vi "Adjust Position.vi"(7 "VI in":refnum<vi>, 8 "error in":errorcluster, 11 "Current Position":T1) -> (0 "error out":errorcluster, 3 "Adjusted Position":T1)   [LabVIEW 2020, in "Editor Position.lvclass"]
doc: "Offsets to current windows bounds in order to prove the window was moved by the VI being tested."
uses:
  Editor Position.lvclass
  Editor Position.lvclass/Editor Position.ctl
  <vilib>/Utility/miscctls.llb/LVRectTypeDef.ctl
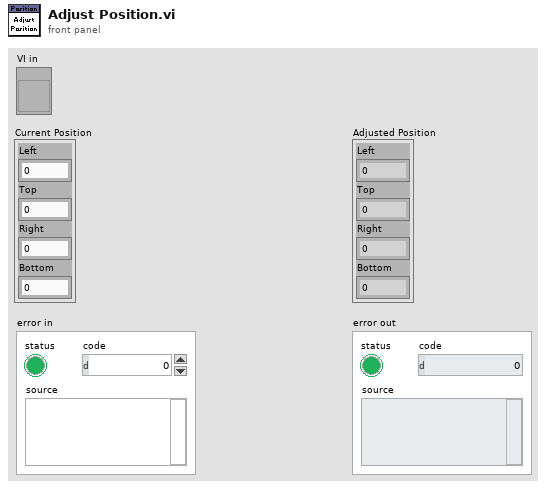
[diagram p1: front panel]
types:
  T1 = typedef "LVRectTypeDef.ctl" = cluster{"Left":i16, "Top":i16, "Right":i16, "Bottom":i16}
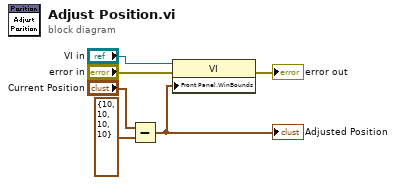
[diagram p0: block diagram]
diagram:
  n1 = Subtract(x="Current Position", y=T1 {"Left"=10, "Top"=10, "Right"=10, "Bottom"=10}) -> (x-y=w1:T1)
  "Adjusted Position" <- w1
  n2 = property class="VI"(reference="VI in", error in="error in", "Front Panel.WinBounds"=w1) -> (error out=→"error out":errorcluster)  [unwired: 1 out]
